vi "Start Step Logger.vi"(8 "error in (no error)":errorcluster, 11 "Measurement in":refnum<class "Measurement.lvclass">) -> (0 "error out":errorcluster, 3 "Measurement out":refnum<class "Measurement.lvclass">)   [LabVIEW 2017, in "Measurement Actor.lvlib" / "Measurement.lvclass"]
uses:
  Measurement.lvclass
  <vilib>/ActorFramework/Actor/Actor.lvclass
  Configuration/Step Configuration.lvclass
  Logger/Logger.lvclass
  Logger/config/Logger Configuration.lvclass
  C:/Program Files (x86)/National Instruments/LabVIEW 2017/vi.lib/ActorFramework/Actor/Actor.lvclass
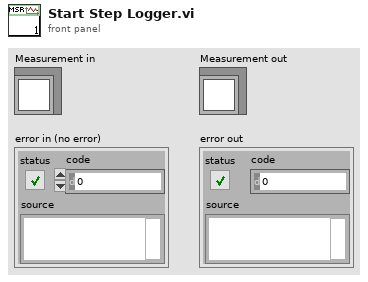
[diagram p1: front panel]
types:
  T1 = cluster{"File Name":string, "Upload Files to SystemLink Server":bool, "Max Samples Per File":i32, "Folder Location":path, "Logging":bool}
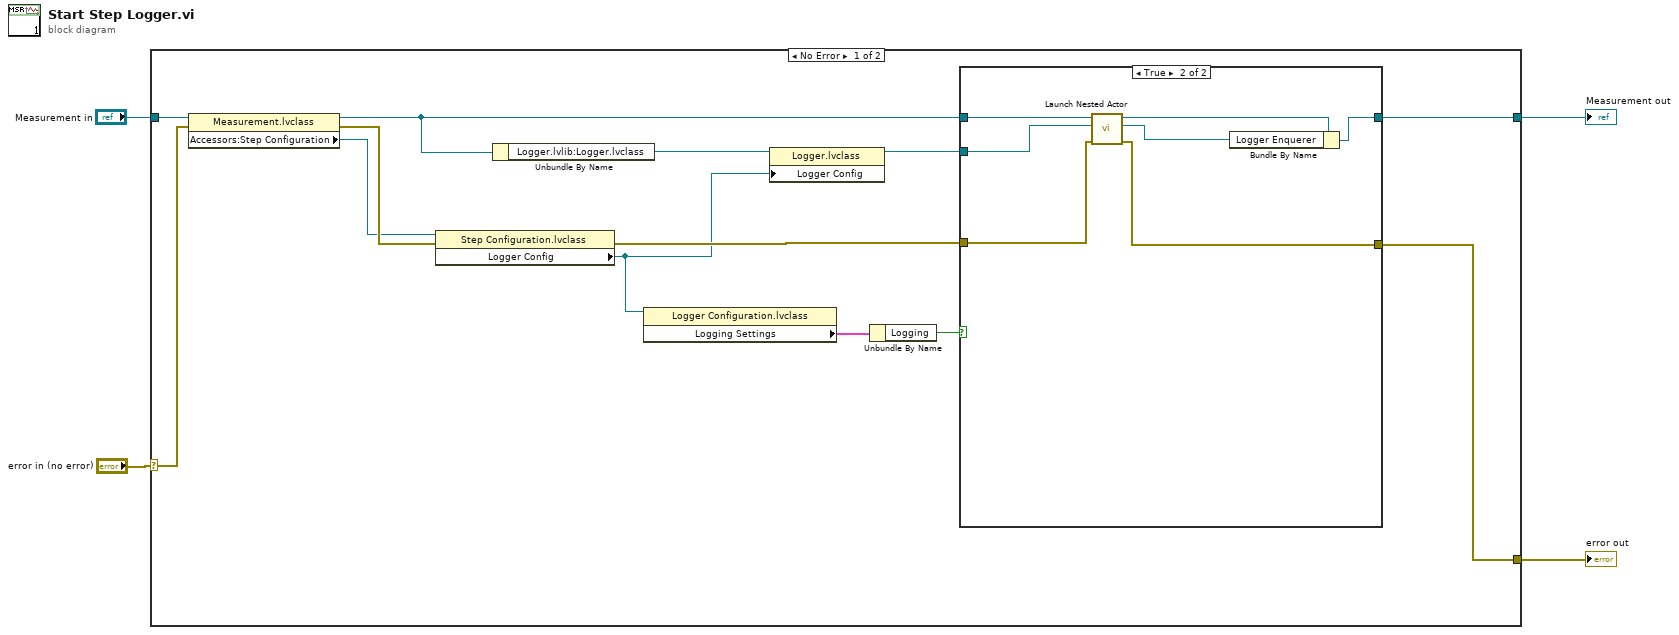
[diagram p0: block diagram]
diagram:
  n1 = case shown="No Error" "error in (no error)" {
    selector: "error in (no error)" -> [w9 w27]
    tunnel: "Measurement in" -> [w15 w28]
    tunnel: [w12 w28] -> w3
    tunnel: [w10 w27] -> w2
    frame No Error {
      n2 = property class="Measurement.lvclass"(reference=w15, error in=w9) -> (reference out=w13:refnum<class "Measurement.lvclass">, error out=w17:errorcluster, "Accessors:Step Configuration"=w16:refnum<class "Step Configuration.lvclass">)
      n3 = property class="Step Configuration.lvclass"(reference=w16, error in=w17) -> (error out=w11:errorcluster, "Logger Config"=w6:refnum<class "Logger Configuration.lvclass">)  [unwired: 1 out]
      n4 = Unbundle By Name(w13) -> ("Logger.lvlib:Logger.lvclass"=w8:refnum<class "Logger.lvclass">)
      n5 = property class="Logger Configuration.lvclass"(reference=w6) -> ("Logging Settings"=w5:T1)  [unwired: 1 in, 2 out]
      n6 = property class="Logger.lvclass"(reference=w8, "Logger Config"=w6) -> (reference out=w7:refnum<class "Logger.lvclass">)  [unwired: 1 in, 1 out]
      n7 = Unbundle By Name(w5) -> ("Logging"=w14:bool)
      n8 = case shown="True" w14 {
        tunnel: w7 -> [_ w25]
        tunnel: w13 -> [w19 w26]
        tunnel: [w19 w21] -> w12
        tunnel: w11 -> [w18 w24]
        tunnel: [w18 w23] -> w10
        frame False {
        }
        frame True {
          n9 = call <vilib>:"Launch Nested Actor.vi"("error in (no error)"=w24, "Nested Actor"=w25, "Caller Actor in"=w26) -> ("error out"=w23:errorcluster, "Nested Actor's Enqueuer"=w20:refnum<class "Message Enqueuer.lvclass">, "Caller Actor out"=w22:refnum<class "Measurement.lvclass">)  [unwired: 6 in]
          n10 = Bundle By Name(cluster=w22, "Logger Enquerer"=w20) -> (w21:refnum<class "Measurement.lvclass">)
        }
      }
    }
    frame Error {
    }
  }
  "error out" <- w2
  "Measurement out" <- w3
